vi "serialcommunication v3.vi"() -> ()   [LabVIEW 2009]
uses:
  <vilib>/Instr/_visa.llb/VISA Configure Serial Port (Instr).vi
panel:
  out "error out":errorcluster
  in  "stop":bool
  in  "write string":string
  in  "write":bool
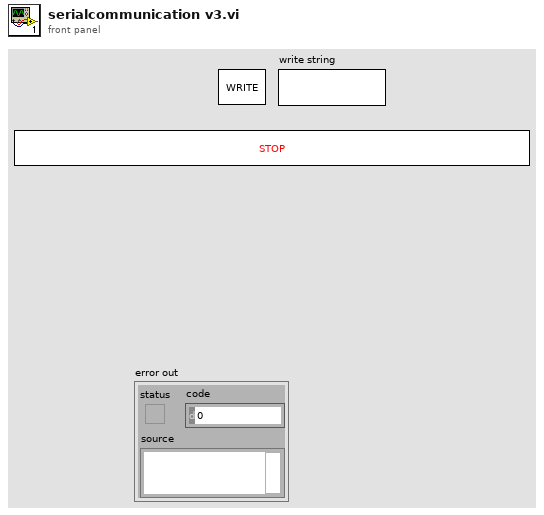
[diagram p1: front panel]
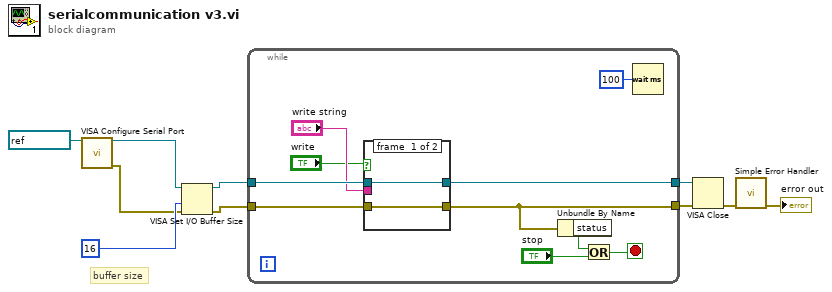
[diagram p0: block diagram]
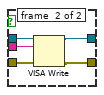
[diagram p2: hidden frame]
diagram:
  # "buffer size"
  n1 = call-poly "VISA Configure Serial Port"("VISA resource name"=refnum<visa-resource-name> "COM3") -> ("VISA resource name out"=w2:refnum<visa-resource-name>, "error out"=w1:errorcluster)  [unwired: 13 in]
  n2 = VISA Set I/O Buffer Size(VISA resource name=w2, size (4096)=u32 16 ("buffer size"), error in (no error)=w1) -> (VISA resource name out=w3:refnum<visa-resource-name>, error out=w4:errorcluster)  [unwired: 1 in]
  n3 = while {
    tunnel: w3 -> [w17]
    tunnel: w4 -> [w16]
    tunnel: [w12] -> w9
    tunnel: [w11] -> w8
    stop <- w18 stop-if-true
    n4 = case shown="True" "write" {
      tunnel: w17 -> [w22 w27]
      tunnel: w16 -> [w21 w26]
      tunnel: [w22 w25] -> w12
      tunnel: [w21 w24] -> w11
      tunnel: "write string" -> [_ w23]
      frame #0 {
      }
      frame #1 {
        n5 = VISA Write(VISA resource name=w27, write buffer=w23, error in (no error)=w26) -> (VISA resource name out=w25:refnum<visa-resource-name>, error out=w24:errorcluster)  [unwired: 1 out]
      }
    }
    n6 = Unbundle By Name(w11) -> ("status"=w20:bool)
    n7 = Or(x=w20, y="stop") -> (x .or. y?=w18:bool)
    n8 = Wait (ms)(milliseconds to wait=u32 100) -> ()  [unwired: 1 out]
  }
  n9 = VISA Close(VISA resource name=w9, error in (no error)=w8) -> (error out=w7:errorcluster)
  n10 = call <vilib>:"Simple Error Handler.vi"("error in (no error)"=w7) -> ("error out"=→"error out":errorcluster)  [unwired: 4 in, 4 out]
